vi "Disconnect.vi"(8 "エラー入力（エラーなし）":errorcluster, 11 "Handler out":T1) -> (0 "エラー出力":errorcluster)   [LabVIEW 2015, in "LV_CloudTranslationAPI.lvlib"]
uses:
  LV_CloudTranslationAPI.lvlib
  Handler.ctl
  <vilib>/httpClient/ClientHandle.ctl
  <vilib>/httpClient/LabVIEWHTTPClient.lvlib
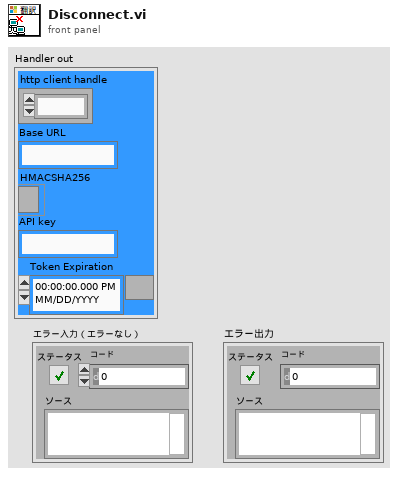
[diagram p1: front panel]
types:
  T1 = typedef "LV_CloudTranslationAPI.lvlib/Handler.ctl" = cluster{"http client handle":T2, "Base URL":string, "HMACSHA256":refnum<k24>, "API key":string, "Token Expiration ":timestamp}
  T2 = typedef "LabVIEWHTTPClient.lvlib/ClientHandle.ctl" = refnum<k1>
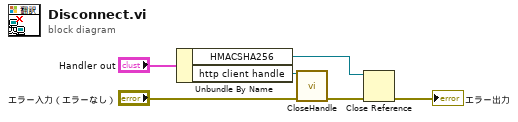
[diagram p0: block diagram]
diagram:
  n1 = Unbundle By Name("Handler out") -> ("HMACSHA256"=w3:refnum<k24>, "http client handle"=w5:T2)
  n2 = call <vilib>:"CloseHandle.vi"("client handle"=w5, "error in (no error)"="エラー入力（エラーなし）") -> ("error out"=w2:errorcluster)  [unwired: 13 in]
  n3 = Close Reference(reference=w3, error in (no error)=w2) -> (error out=→"エラー出力":errorcluster)
